vi "Specs.vi"() -> ()   [LabVIEW 2017]
uses:
  controls/All Specs.ctl
  controls/Specifications.ctl
panel:
  in  "Post Flash":bool
  in  "Pre flash":bool
  in  "Shipping":dbl=86.0
  out "Stall Test?":bool
  in  "All Specs":T1={"LH"={"Go Up"={"Min Speed"=0.0, "Max Speed"=0.0, "Min Time"=0.0, "Max Time"=0.0, "Min Run Current"=0.0, "Max Run Current"=10.0, "Min Stall Current"=0.0, "Max Stall Current"=0.0, "Min Stall Force"=170.0, "Max Stall Force"=320.0, "Min Stroke"=254.4, "Max Stroke"=270.4}, "Go Down"={"Min Speed"=0.0, "Max Speed"=0.0, "Min Travel Time"=0.0, "Max Travel Time"=0.0, "Min Run Current"=0.0, "Max Run Current"=10.0}, "Shipping"={"Min Distance"=0.0, "Max Distance"=0.0, "Setpoint"=5.0}, "Anti-Pinch"={"Min Force"=5.0, "Max Force"=15.0}}, "RH"={"Go Up"={"Min Speed"=0.0, "Max Speed"=0.0, "Min Time"=0.0, "Max Time"=0.0, "Min Run Current"=0.0, "Max Run Current"=10.0, "Min Stall Current"=0.0, "Max Stall Current"=0.0, "Min Stall Force"=170.0, "Max Stall Force"=320.0, "Min Stroke"=254.4, "Max Stroke"=270.4}, "Go Down"={"Min Speed"=0.0, "Max Speed"=0.0, "Min Travel Time"=0.0, "Max Travel Time"=0.0, "Min Run Current"=0.0, "Max Run Current"=10.0}, "Shipping"={"Min Distance"=0.0, "Max Distance"=0.0, "Setpoint"=5.0}, "Anti-Pinch"={"Min Force"=5.0, "Max Force"=15.0}}, "W 601 FR RH Std"={"Go Up"={"Min Speed"=10.0, "Max Speed"=250.0, "Min Time"=0.5, "Max Time"=4.3, "Min Run Current"=0.0, "Max Run Current"=10.0, "Min Stall Current"=0.0, "Max Stall Current"=25.0, "Min Stall Force"=170.0, "Max Stall Force"=320.0, "Min Stroke"=254.4, "Max Stroke"=270.4}, "Go Down"={"Min Speed"=10.0, "Max Speed"=250.0, "Min Travel Time"=0.5, "Max Travel Time"=4.3, "Min Run Current"=0.0, "Max Run Current"=10.0}, "Shipping"={"Min Distance"=5.0, "Max Distance"=15.0, "Setpoint"=5.0}, "Anti-Pinch"={"Min Force"=5.0, "Max Force"=15.0}}, "W 601 FR LH Std"={"Go Up"={"Min Speed"=10.0, "Max Speed"=250.0, "Min Time"=0.5, "Max Time"=4.3, "Min Run Current"=0.0, "Max Run Current"=10.0, "Min Stall Current"=0.0, "Max Stall Current"=25.0, "Min Stall Force"=170.0, "Max Stall Force"=320.0, "Min Stroke"=254.4, "Max Stroke"=270.4}, "Go Down"={"Min Speed"=10.0, "Max Speed"=250.0, "Min Travel Time"=0.5, "Max Travel Time"=4.3, "Min Run Current"=0.0, "Max Run Current"=10.0}, "Shipping"={"Min Distance"=5.0, "Max Distance"=15.0, "Setpoint"=5.0}, "Anti-Pinch"={"Min Force"=5.0, "Max Force"=15.0}}, "W 601 RR RH Std"={"Go Up"={"Min Speed"=10.0, "Max Speed"=250.0, "Min Time"=0.5, "Max Time"=4.3, "Min Run Current"=0.0, "Max Run Current"=10.0, "Min Stall Current"=0.0, "Max Stall Current"=25.0, "Min Stall Force"=170.0, "Max Stall Force"=320.0, "Min Stroke"=254.4, "Max Stroke"=270.4}, "Go Down"={"Min Speed"=10.0, "Max Speed"=250.0, "Min Travel Time"=0.5, "Max Travel Time"=4.3, "Min Run Current"=0.0, "Max Run Current"=10.0}, "Shipping"={"Min Distance"=5.0, "Max Distance"=15.0, "Setpoint"=5.0}, "Anti-Pinch"={"Min Force"=5.0, "Max Force"=15.0}}, "W 601 RR LH Std"={"Go Up"={"Min Speed"=10.0, "Max Speed"=250.0, "Min Time"=0.5, "Max Time"=4.3, "Min Run Current"=0.0, "Max Run Current"=10.0, "Min Stall Current"=0.0, "Max Stall Current"=25.0, "Min Stall Force"=170.0, "Max Stall Force"=320.0, "Min Stroke"=254.4, "Max Stroke"=270.4}, "Go Down"={"Min Speed"=10.0, "Max Speed"=250.0, "Min Travel Time"=0.5, "Max Travel Time"=4.3, "Min Run Current"=0.0, "Max Run Current"=10.0}, "Shipping"={"Min Distance"=5.0, "Max Distance"=15.0, "Setpoint"=5.0}, "Anti-Pinch"={"Min Force"=5.0, "Max Force"=15.0}}, "W 601 FR RH AP"={"Go Up"={"Min Speed"=10.0, "Max Speed"=250.0, "Min Time"=0.5, "Max Time"=4.3, "Min Run Current"=0.0, "Max Run Current"=10.0, "Min Stall Current"=0.0, "Max Stall Current"=25.0, "Min Stall Force"=170.0, "Max Stall Force"=320.0, "Min Stroke"=254.4, "Max Stroke"=270.4}, "Go Down"={"Min Speed"=10.0, "Max Speed"=250.0, "Min Travel Time"=0.5, "Max Travel Time"=4.3, "Min Run Current"=0.0, "Max Run Current"=10.0}, "Shipping"={"Min Distance"=5.0, "Max Distance"=15.0, "Setpoint"=5.0}, "Anti-Pinch"={"Min Force"=5.0, "Max Force"=15.0}}, "W 601 FR LH AP"={"Go Up"={"Min Speed"=10.0, "Max Speed"=250.0, "Min Time"=0.5, "Max Time"=4.3, "Min Run Current"=0.0, "Max Run Current"=10.0, "Min Stall Current"=0.0, "Max Stall Current"=25.0, "Min Stall Force"=170.0, "Max Stall Force"=320.0, "Min Stroke"=254.4, "Max Stroke"=270.4}, "Go Down"={"Min Speed"=10.0, "Max Speed"=250.0, "Min Travel Time"=0.5, "Max Travel Time"=4.3, "Min Run Current"=0.0, "Max Run Current"=10.0}, "Shipping"={"Min Distance"=5.0, "Max Distance"=15.0, "Setpoint"=5.0}, "Anti-Pinch"={"Min Force"=5.0, "Max Force"=15.0}}, "W 601 RR RH AP"={"Go Up"={"Min Speed"=10.0, "Max Speed"=250.0, "Min Time"=0.5, "Max Time"=4.3, "Min Run Current"=0.0, "Max Run Current"=10.0, "Min Stall Current"=0.0, "Max Stall Current"=25.0, "Min Stall Force"=170.0, "Max Stall Force"=320.0, "Min Stroke"=254.4, "Max Stroke"=270.4}, "Go Down"={"Min Speed"=10.0, "Max Speed"=250.0, "Min Travel Time"=0.5, "Max Travel Time"=4.3, "Min Run Current"=0.0, "Max Run Current"=10.0}, "Shipping"={"Min Distance"=5.0, "Max Distance"=15.0, "Setpoint"=5.0}, "Anti-Pinch"={"Min Force"=5.0, "Max Force"=15.0}}, "W 601 RR LH AP"={"Go Up"={"Min Speed"=10.0, "Max Speed"=250.0, "Min Time"=0.5, "Max Time"=4.3, "Min Run Current"=0.0, "Max Run Current"=10.0, "Min Stall Current"=0.0, "Max Stall Current"=25.0, "Min Stall Force"=170.0, "Max Stall Force"=320.0, "Min Stroke"=254.4, "Max Stroke"=270.4}, "Go Down"={"Min Speed"=10.0, "Max Speed"=250.0, "Min Travel Time"=0.5, "Max Travel Time"=4.3, "Min Run Current"=0.0, "Max Run Current"=10.0}, "Shipping"={"Min Distance"=5.0, "Max Distance"=15.0, "Setpoint"=5.0}, "Anti-Pinch"={"Min Force"=5.0, "Max Force"=15.0}}}
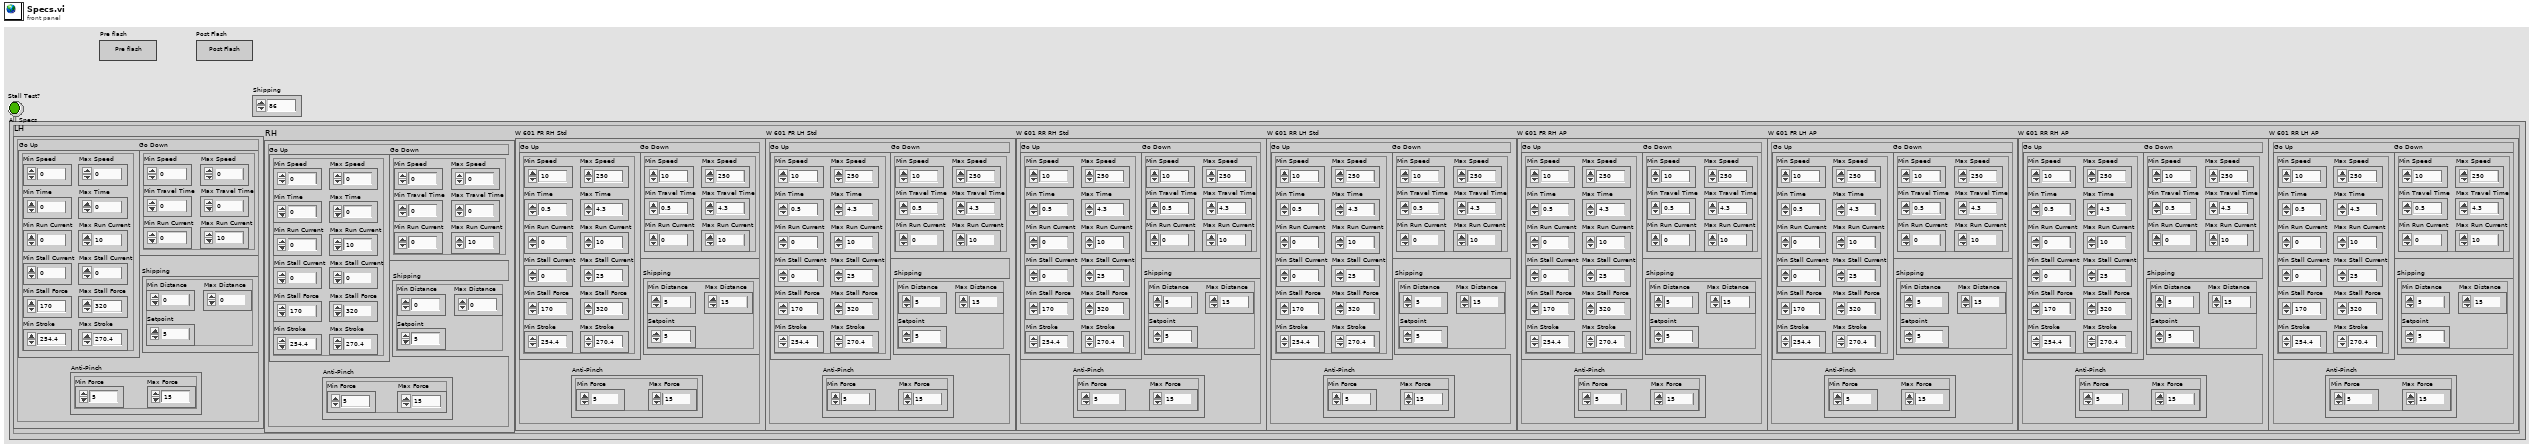
[diagram p1: front panel]
types:
  T1 = typedef "All Specs.ctl" = cluster{"LH":T2, "RH":T2, "W 601 FR RH Std":T2, "W 601 FR LH Std":T2, "W 601 RR RH Std":T2, "W 601 RR LH Std":T2, "W 601 FR RH AP":T2, "W 601 FR LH AP":T2, "W 601 RR RH AP":T2, "W 601 RR LH AP":T2}
  T2 = typedef "Specifications.ctl" = cluster{"Go Up":cluster{"Min Speed":dbl, "Max Speed":dbl, "Min Time":dbl, "Max Time":dbl, "Min Run Current":dbl, "Max Run Current":dbl, "Min Stall Current":dbl, "Max Stall Current":dbl, "Min Stall Force":dbl, "Max Stall Force":dbl, "Min Stroke":dbl, "Max Stroke":dbl}, "Go Down":cluster{"Min Speed":dbl, "Max Speed":dbl, "Min Travel Time":dbl, "Max Travel Time":dbl, "Min Run Current":dbl, "Max Run Current":dbl}, "Shipping":cluster{"Min Distance":dbl, "Max Distance":dbl, "Setpoint":dbl}, "Anti-Pinch":cluster{"Min Force":dbl, "Max Force":dbl}}
diagram:
